vi "RCMEditor.vi"() -> ()   [LabVIEW 2020]
uses:
  <vilib>/Utility/miscctls.llb/LVSelectionTypeDef.ctl
  Type Definitions/RCMControlStatus.ctl
  Support/Tree Control/Library/TreeControl.lvclass
  Support/Refnum/Library/Refnum.lvlib
panel:
  in  "item type":string(combo)="User" caption="Item Type:"
  in  "btn1: exit":bool
  in  "btn1: save as":bool
  in  "btn1: save":bool
  in  "btn1: open":bool
  in  "btn1: new":bool
  in  "item icon path":path caption="Item ICON Path:"
  in  "item name":string caption="Item Name:"
  in  "btn2: down":bool
  in  "btn2: up":bool
  in  "btn2: indent":bool
  in  "btn2: outdent":bool
  in  "btn2: delete":bool
  in  "btn2: add":bool
  in  "tree":string(tree)
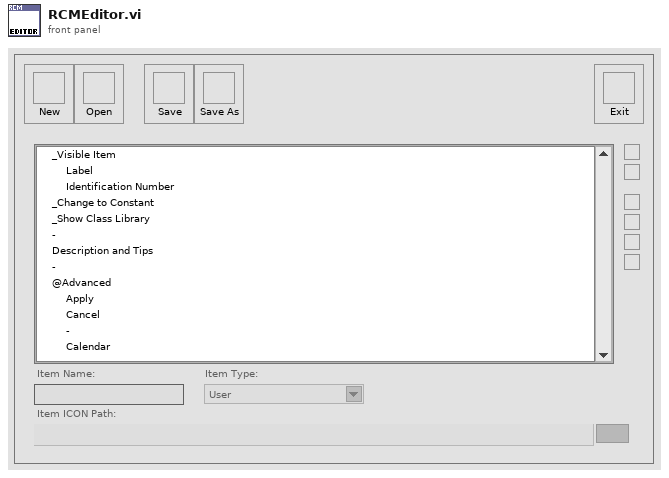
[diagram p1: front panel]
types:
  T1 = typedef "LVSelectionTypeDef.ctl" = cluster{"Selection Start":u32, "Selection End":u32}
  T2 = typedef "RCMControlStatus.ctl" = enum16{"disable all", "initialize", "enable save", "disable save", "enable tree edit", "disable tree edit", "enable item edit", "disable item edit", "user", "seperator"}
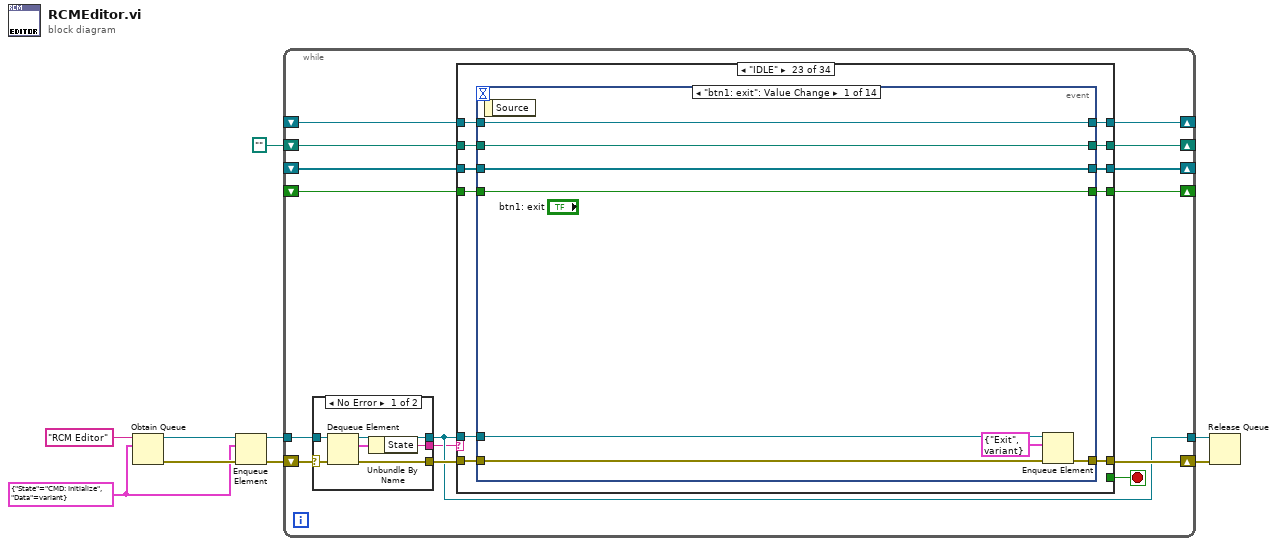
[diagram p0: block diagram]
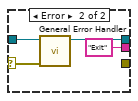
[diagram p2: hidden frame]
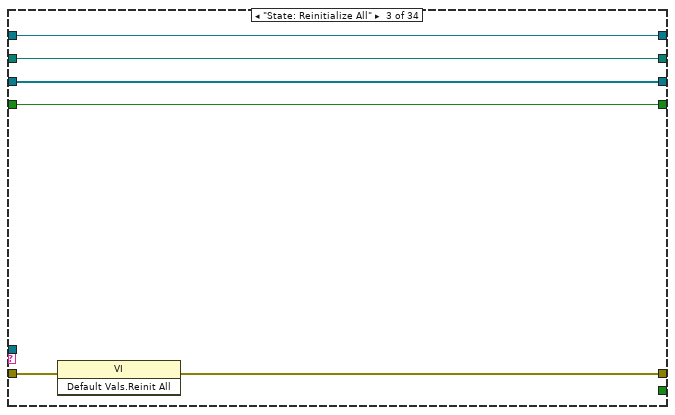
[diagram p5: hidden frame]
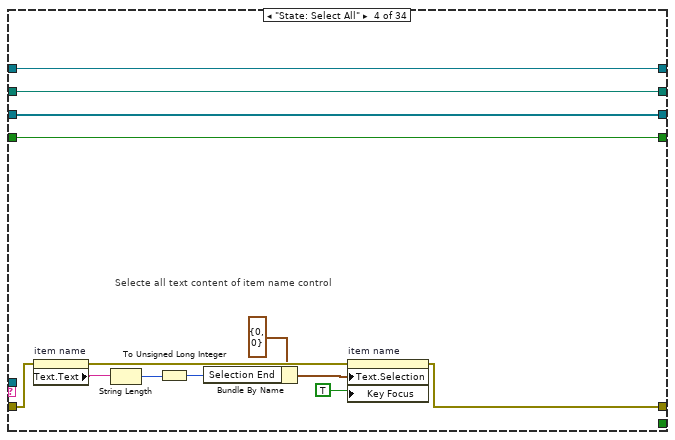
[diagram p6: hidden frame]
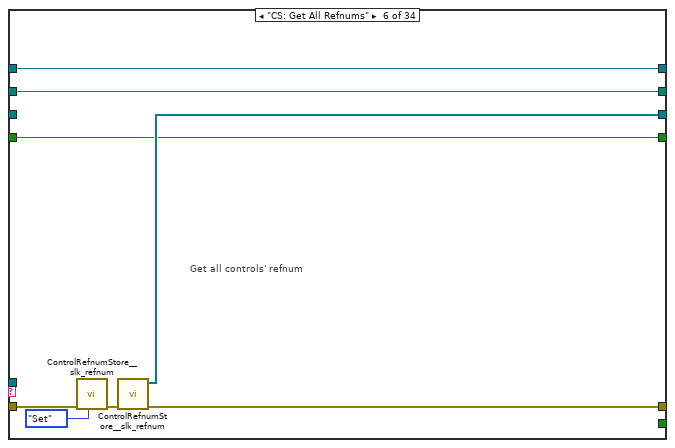
[diagram p8: hidden frame]
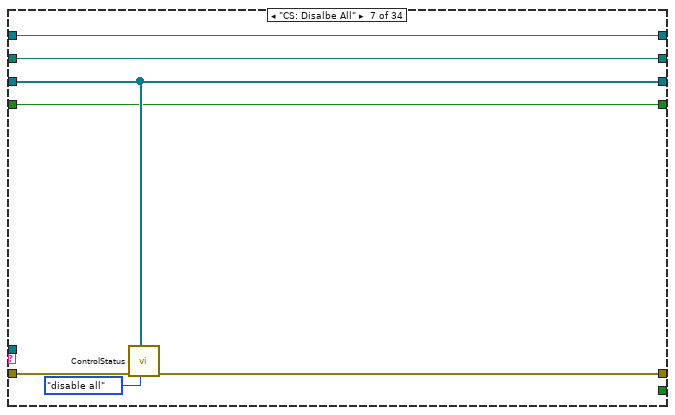
[diagram p9: hidden frame]
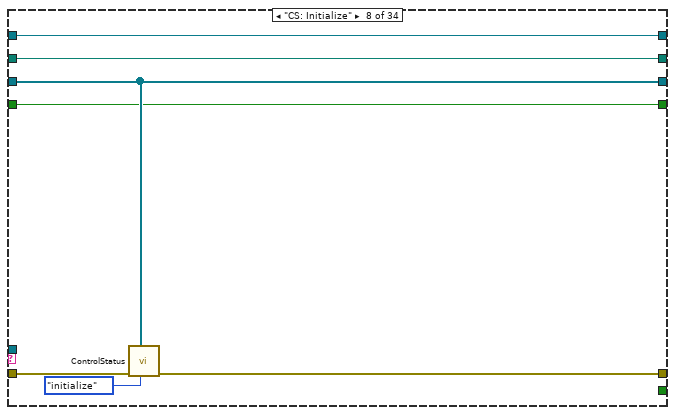
[diagram p10: hidden frame]
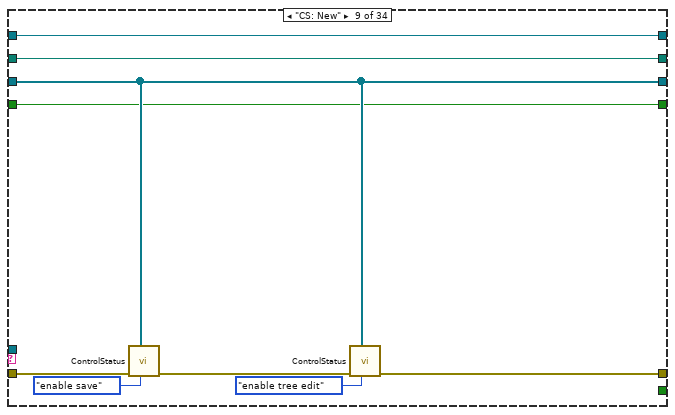
[diagram p11: hidden frame]
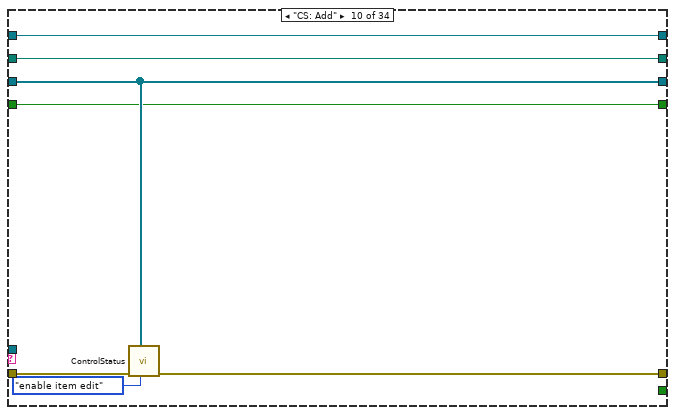
[diagram p12: hidden frame]
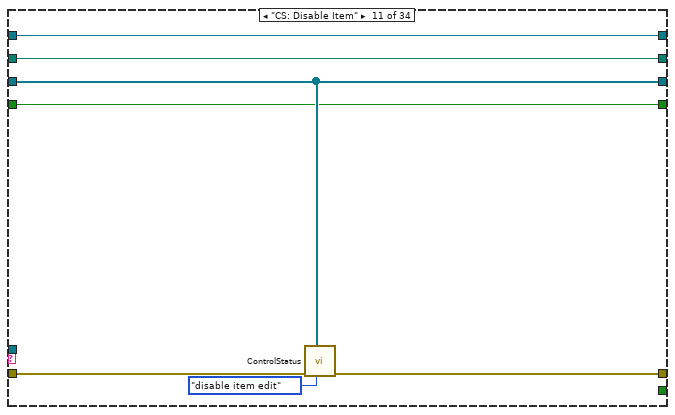
[diagram p13: hidden frame]
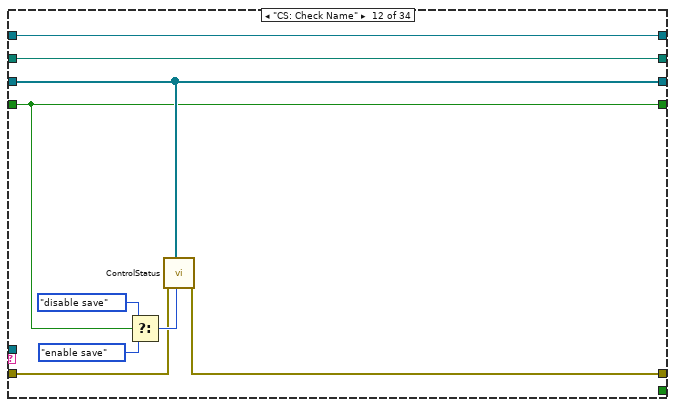
[diagram p14: hidden frame]
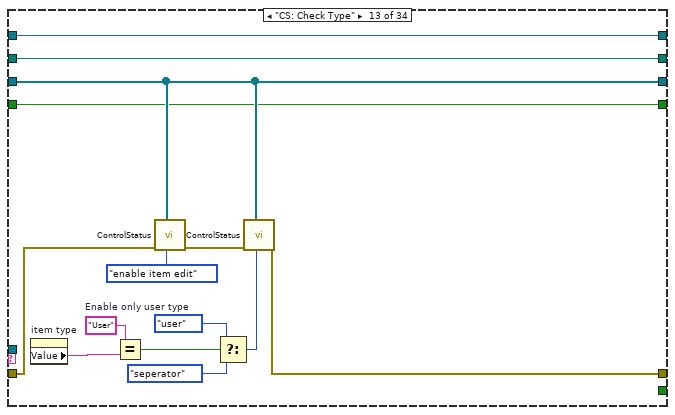
[diagram p15: hidden frame]
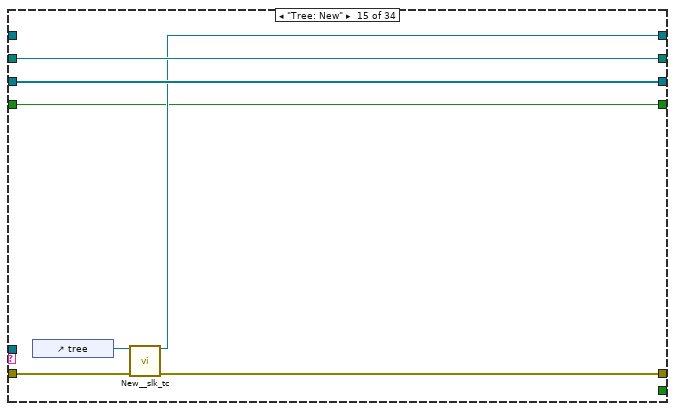
[diagram p17: hidden frame]
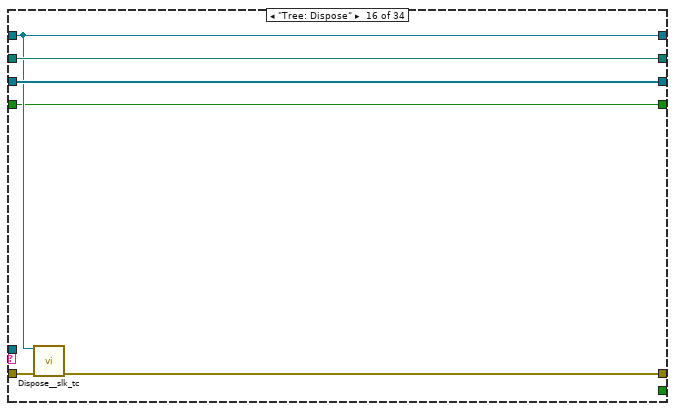
[diagram p18: hidden frame]
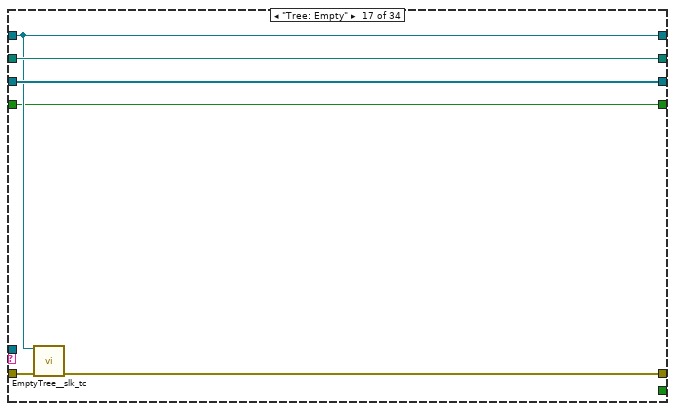
[diagram p19: hidden frame]
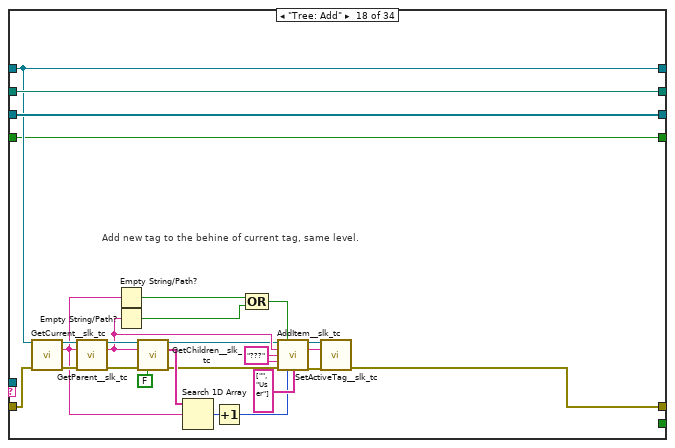
[diagram p20: hidden frame]
diagram:
  w2 = cluster{"State":string, "Data":variant} {"State"="CMD: Initialize", "Data"=variant}
  n1 = Obtain Queue(name (unnamed)="RCM Editor", element data type=w2) -> (queue out=w8:refnum<queue>, error out=w7:errorcluster)  [unwired: 3 in, 1 out]
  n2 = Enqueue Element(queue=w8, element=w2, error in (no error)=w7) -> (queue out=w4:refnum<queue>, error out=w3:errorcluster)  [unwired: 2 out]
  n3 = while {
    tunnel: w4 -> [w23]
    shift-right: [w21] -> w5
    shift-left: w3 -> [w24]
    shift-right: [w19] -> _
    shift-left: _ -> [w20]
    shift-right: [w15] -> _
    shift-left: path "" -> [w18]
    shift-right: [w16] -> _
    shift-left: _ -> [w17]
    tunnel: [w14] -> w6
    shift-right: [w11] -> _
    shift-left: _ -> [w10]
    stop <- w13 stop-if-true
    n4 = case shown="No Error" w24 {
      selector: w24 -> [w29 w33]
      tunnel: w23 -> [w30 w32]
      tunnel: [w25 "Exit" ("State")] -> w12
      tunnel: [w27 _] -> w22
      tunnel: [w26 w32] -> w14
      frame No Error {
        n5 = Dequeue Element(queue=w30, error in (no error)=w29) -> (queue out=w26:refnum<queue>, element=w28:cluster{"State":string, "Data":variant}, error out=w27:errorcluster)  [unwired: 2 out]
        n6 = Unbundle By Name(w28) -> ("State"=w25:string)
      }
      frame Error {
        n7 = call <vilib>:"General Error Handler.vi"("error in (no error)"=w33) -> ()  [unwired: 2 in, 13 out]
      }
    }
    n8 = case shown="\"IDLE\"" w12 {
      tunnel: w22 -> [w38 w43 w49 w62 w64 w72 w80 w87 w96 w103 w110 w114 w124 w140 w145 w151 w159 w173 w202 w209 w225 w242 w252 w387 w395 w407 w419 w431 w443 w455 w467 w479 w488 w491]
      tunnel: [w38 w43 w45 w50 w64 w71 w77 w84 w94 w100 w107 w113 w127 w140 w144 w150 w156 w160 w194 w206 w224 w242 w251 w387 w391 w403 w415 w427 w439 w451 w463 w475 w488 w491] -> w21
      tunnel: w14 -> [_ _ _ _ _ _ _ _ _ _ _ _ _ _ _ _ _ _ _ _ _ _ w253 _ w390 w402 w414 w426 w438 w450 w462 w474 _ _]
      tunnel: w20 -> [w37 w42 w48 w61 w67 w75 w82 w89 w98 w105 w112 w121 w128 w139 _ w149 w155 w172 w203 w208 w227 w241 w250 w386 w394 w406 w418 w430 w442 w454 w466 w478 w487 w494]
      tunnel: [w37 w42 w48 w61 w67 w75 w82 w89 w98 w105 w112 w121 w128 w139 w142 w149 w155 w172 w203 w208 w227 w241 w249 w386 w394 w406 w418 w430 w442 w454 w466 w478 w487 w494] -> w19
      tunnel: w18 -> [w35 w40 w47 w60 w66 w74 w81 w88 w97 w104 w111 w120 w135 w137 w146 w152 w157 w185 w204 w216 w237 w239 w248 w384 w392 w404 w416 w428 w440 w452 w464 w476 w485 w492]
      tunnel: w17 -> [w36 w41 w46 w59 w65 _ w79 w86 w93 w102 w109 w116 w125 w138 w147 w153 w158 w184 w205 w210 w226 w240 w247 w385 w393 w405 w417 w429 w441 w453 w465 w477 w486 w493]
      tunnel: [w36 w41 w46 w59 w65 w70 w79 w86 w93 w102 w109 w116 w125 w138 w147 w153 w158 w184 w205 w210 w226 w240 w246 w385 w393 w405 w417 w429 w441 w453 w465 w477 w486 w493] -> w16
      tunnel: [w35 w40 w47 w60 w66 w74 w81 w88 w97 w104 w111 w120 w135 w137 w146 w152 w157 w185 w204 w216 w237 w239 w245 w384 w392 w404 w416 w428 w440 w452 w464 w476 w485 w492] -> w15
      tunnel: [_ _ _ _ _ _ _ _ _ _ _ _ _ _ _ _ _ _ _ _ _ _ _ _ _ _ _ _ _ _ _ _ _ TRUE] -> w13
      tunnel: [w34 w39 w44 w58 w63 w68 w76 w83 w90 w99 w106 w115 w122 w136 w141 w148 w154 w161 w191 w207 w223 w238 w243 w383 w388 w400 w412 w424 w436 w448 w460 w472 w484 w489] -> w11
      tunnel: w10 -> [w34 w39 w44 w58 w63 w68 w76 w83 w90 w99 w106 w115 w122 w136 w141 w148 w154 w161 w191 _ w223 w238 w244 w383 w388 w400 w412 w424 w436 w448 w460 w472 w484 w489]
      frame Default {
      }
      frame "----State----" {
      }
      frame "State: Reinitialize All" {
        n9 = invoke class="VI" method="Default Vals.Reinit All"(error in=w49) -> (error out=w45:errorcluster)  [unwired: 2 in, 2 out]
      }
      frame "State: Select All" {
        # "Selecte all text content of item name control"
        n10 = property on="item name" class="Str"(error in=w62) -> (error out=w57:errorcluster, "Text.Text"=w53:string)  [unwired: 1 in, 1 out]
        n11 = String Length(string=w53) -> (length=w52:i32)
        n12 = To Unsigned Long Integer(number=w52) -> (unsigned 32bit integer=w51:u32)
        n13 = Bundle By Name(cluster=T1 {"Selection Start"=0, "Selection End"=0} ("Text.Selection"), "Selection End"=w51) -> (w54:T1)
        n14 = property on="item name" class="Str"(error in=w57, "Text.Selection"=w54, "Key Focus"=TRUE) -> (error out=w50:errorcluster)  [unwired: 1 in, 1 out]
      }
      frame "----Control Status----" {
      }
      frame "CS: Get All Refnums" {
        # "Get all controls' refnum"
        n15 = call "ControlRefnumStore__slk_refnum.vi"("cmd (Get)"=enum16{"Set", "Get"}."Set", "error in (no error)"=w72) -> ("error out"=w73:errorcluster)  [unwired: 8 in, 1 out]
        n16 = call "ControlRefnumStore__slk_refnum.vi"("error in (no error)"=w73) -> ("error out"=w71:errorcluster, "control refnum array out"=w70:refnum<vi>[])  [unwired: 9 in]
      }
      frame "CS: Disalbe All" {
        n17 = call "ControlStatus.vi"("state"=RCMControlStatus."disable all", "control refnum array in"=w79, "error in (no error)"=w80) -> ("error out"=w77:errorcluster)  [unwired: 8 in]
      }
      frame "CS: Initialize" {
        n18 = call "ControlStatus.vi"("state"=RCMControlStatus."initialize", "control refnum array in"=w86, "error in (no error)"=w87) -> ("error out"=w84:errorcluster)  [unwired: 8 in]
      }
      frame "CS: New" {
        n19 = call "ControlStatus.vi"("state"=RCMControlStatus."enable save", "control refnum array in"=w93, "error in (no error)"=w96) -> ("error out"=w95:errorcluster)  [unwired: 8 in]
        n20 = call "ControlStatus.vi"("state"=RCMControlStatus."enable tree edit", "control refnum array in"=w93, "error in (no error)"=w95) -> ("error out"=w94:errorcluster)  [unwired: 8 in]
      }
      frame "CS: Add" {
        n21 = call "ControlStatus.vi"("state"=RCMControlStatus."enable item edit", "control refnum array in"=w102, "error in (no error)"=w103) -> ("error out"=w100:errorcluster)  [unwired: 8 in]
      }
      frame "CS: Disable Item" {
        n22 = call "ControlStatus.vi"("state"=RCMControlStatus."disable item edit", "control refnum array in"=w109, "error in (no error)"=w110) -> ("error out"=w107:errorcluster)  [unwired: 8 in]
      }
      frame "CS: Check Name" {
        n23 = Select(t=RCMControlStatus."disable save" ("state"), s=w115, f=RCMControlStatus."enable save" ("state")) -> (s? t:f=w117:T2)
        n24 = call "ControlStatus.vi"("state"=w117, "control refnum array in"=w116, "error in (no error)"=w114) -> ("error out"=w113:errorcluster)  [unwired: 8 in]
      }
      frame "CS: Check Type" {
        w133 = "User"  # Enable only user type
        n25 = property on="item type" class="CmbBox"() -> ("Value"=w134:string)  [unwired: 2 in, 2 out]
        n26 = Equal?(x=w133, y=w134) -> (x = y?=w129:bool)
        n27 = call "ControlStatus.vi"("state"=RCMControlStatus."enable item edit", "control refnum array in"=w125, "error in (no error)"=w124) -> ("error out"=w123:errorcluster)  [unwired: 8 in]
        n28 = Select(t=RCMControlStatus."user" ("state"), s=w129, f=RCMControlStatus."seperator" ("state")) -> (s? t:f=w130:T2)
        n29 = call "ControlStatus.vi"("state"=w130, "control refnum array in"=w125, "error in (no error)"=w123) -> ("error out"=w127:errorcluster)  [unwired: 8 in]
      }
      frame "----Tree----" {
      }
      frame "Tree: New" {
        n30 = control-ref of="tree"() -> (w143:refnum<vi>)
        n31 = call "New__slk_tc.vi"("tree refnum"=w143, "error in (no error)"=w145) -> ("tree control out"=w142:refnum<class "TreeControl.lvclass">, "error out"=w144:errorcluster)  [unwired: 12 in]
      }
      frame "Tree: Dispose" {
        n32 = call "Dispose__slk_tc.vi"("tree control in"=w149, "error in (no error)"=w151) -> ("error out"=w150:errorcluster)  [unwired: 13 in]
      }
      frame "Tree: Empty" {
        n33 = call "EmptyTree__slk_tc.vi"("tree control in"=w155, "error in (no error)"=w159) -> ("error out"=w156:errorcluster)  [unwired: 11 in, 2 out]
      }
      frame "Tree: Add" {
        w178 = "???" ("new tag (same as text)")
        # "Add new tag to the behine of current tag, same level."
        n34 = call "GetCurrent__slk_tc.vi"("tree control in"=w172, "error in (no error)"=w173) -> ("tree control out"=w183:refnum<class "TreeControl.lvclass">, "current tag"=w168:string, "error out"=w181:errorcluster)  [unwired: 10 in, 1 out]
        n35 = call "GetParent__slk_tc.vi"("tree control in"=w183, "child tag (\"\")"=w168, "error in (no error)"=w181) -> ("tree control out"=w171:refnum<class "TreeControl.lvclass">, "parent tag"=w170:string, "error out"=w163:errorcluster)  [unwired: 9 in, 1 out]
        n36 = Empty String/Path?(string/path=w168) -> (empty?=w182:bool)
        n37 = Empty String/Path?(string/path=w170) -> (empty?=w179:bool)
        n38 = call "GetChildren__slk_tc.vi"("tree control in"=w171, "parent tag (\"\")"=w170, "error in (no error)"=w163, "use current (T)"=FALSE) -> ("tree control out"=w164:refnum<class "TreeControl.lvclass">, "children tags"=w169:string[], "error out"=w162:errorcluster)  [unwired: 9 in]
        n39 = Search 1D Array(1D array=w169, element=w168) -> (index of element=w167:i32)  [unwired: 1 in]
        n40 = Increment(x=w167) -> (x+1=w165:i32)
        n41 = Compound Arithmetic op=OR(w182, w179) -> (w180:bool)
        n42 = call "AddItem__slk_tc.vi"("tree control in"=w164, "make top level? (F)"=w180, "parent tag (current tag)"=w170, "new tag (same as text)"=w178, "new text"=w178, "error in (no error)"=w162, "child position (end=-1)"=w165, "column text {#1 and greater} (empty)"=string[] ["", "User"]) -> ("tree control out"=w177:refnum<class "TreeControl.lvclass">, "created tag"=w176:string, "error out"=w175:errorcluster)  [unwired: 5 in]
        n43 = call "SetActiveTag__slk_tc.vi"("tree control in"=w177, "active tag"=w176, "error in (no error)"=w175) -> ("error out"=w160:errorcluster)  [unwired: 11 in, 1 out]
      }
      frame "Tree: Get Value" {
        # "Ignore default value \"???\""
        n44 = call "GetCurrent__slk_tc.vi"("tree control in"=w203, "error in (no error)"=w202) -> ("tree control out"=w201:refnum<class "TreeControl.lvclass">, "current text"=w188:string, "error out"=w198:errorcluster)  [unwired: 10 in, 1 out]
        n45 = Not Equal?(x=w188, y="???" ("x")) -> (x != y?=w190:bool)
        n46 = call "GetCurrent__slk_tc.vi"("tree control in"=w201, "error in (no error)"=w198, "column # (0)"=1) -> ("tree control out"=w200:refnum<class "TreeControl.lvclass">, "current text"=w196:string, "error out"=w197:errorcluster)  [unwired: 9 in, 1 out]
        n47 = Select(t=w188, s=w190, f="") -> (s? t:f=w186:string)
        n48 = String To Path(string=w196) -> (path=w195:path)
        n49 = property on="item name" class="Str"("Value"=w186) -> ()  [unwired: 2 in, 2 out]
        n50 = property on="item icon path" class="Path"("Value"=w195) -> ()  [unwired: 2 in, 2 out]
        n51 = call "GetCurrent__slk_tc.vi"("tree control in"=w200, "error in (no error)"=w197, "column # (0)"=2) -> ("current text"=w193:string, "error out"=w194:errorcluster)  [unwired: 9 in, 2 out]
        n52 = property on="item type" class="CmbBox"("Value"=w193) -> ()  [unwired: 2 in, 2 out]
      }
      frame "Tree: Check Name" {
        # "Check if there are duplicated item name."
        n53 = call "GetAll__slk_tc.vi"("tree control in"=w208, "error in (no error)"=w209) -> ("tree control out"=w215:refnum<class "TreeControl.lvclass">, "output tree items"=w213:string[], "error out"=w214:errorcluster)  [unwired: 10 in, 1 out]
        n54 = for {
          shift-right: [w221] -> _
          shift-left: w215 -> [w222]
          tunnel: [w220] -> w212 mode=indexing
          tunnel: w213 -> [w218] mode=indexing
          shift-right: [w217] -> w211
          shift-left: w214 -> [w219]
          n55 = call "ConvertTag__slk_tc.vi"("tree control in"=w222, "input tag (current tag)"=w218, "error in (no error)"=w219) -> ("tree control out"=w221:refnum<class "TreeControl.lvclass">, "text"=w220:string, "error out"=w217:errorcluster)  [unwired: 9 in, 1 out]
        }
        n56 = call "CheckName.vi"("error in (no error)"=w211, "input array"=w212) -> ("error out"=w206:errorcluster, "duplicated?"=w207:bool)  [unwired: 8 in]
      }
      frame "Tree: Type Change" {
        n57 = call "EditItem__slk_tc.vi"("tree control in"=w227, "new text"="-", "error in (no error)"=w225) -> ("tree control out"=w235:refnum<class "TreeControl.lvclass">, "error out"=w234:errorcluster)  [unwired: 11 in]
        n58 = call "EditItem__slk_tc.vi"("tree control in"=w235, "new text"="", "error in (no error)"=w234, "column # (0)"=1) -> ("tree control out"=w231:refnum<class "TreeControl.lvclass">, "error out"=w230:errorcluster)  [unwired: 10 in]
        n59 = property on="item type" class="CmbBox"() -> ("Value"=w228:string)  [unwired: 2 in, 2 out]
        n60 = call "EditItem__slk_tc.vi"("tree control in"=w231, "new text"=w228, "error in (no error)"=w230, "column # (0)"=2) -> ("error out"=w224:errorcluster)  [unwired: 10 in, 1 out]
      }
      frame "----Event----" {
      }
      frame "IDLE" {
        n61 = event shown="[0] \"btn1: exit\": Value Change" {
          selector: _ -> [_ _ _ _ _ _ _ _ _ _ _ _ _ _]
          dyn-events: _ -> [_ _ _ _ _ _ _ _ _ _ _ _ _ _]
          timeout: _ -> [_ _ _ _ _ _ _ _ _ _ _ _ _ _]
          tunnel: w253 -> [w256 w264 w271 w283 w292 w301 w310 w319 w327 w342 w351 w362 w372 w381]
          tunnel: w252 -> [w257 w265 w272 w280 w289 w298 w307 w316 w324 w333 w347 w358 w368 w375]
          tunnel: [w261 w269 w277 w286 w295 w304 w313 w322 w330 w345 w353 w363 w373 w382] -> w251
          tunnel: w250 -> [w260 w268 w273 w281 w290 w299 w308 w317 w325 w335 w349 w359 w369 w378]
          tunnel: [w260 w268 w273 w281 w290 w299 w308 w317 w325 w335 w349 w359 w369 w378] -> w249
          tunnel: w248 -> [w259 w267 w276 w285 w294 w303 w312 w321 w329 w344 w352 w356 _ _]
          tunnel: w247 -> [w258 w266 w275 w284 w293 w302 w311 w320 w328 w343 w348 w360 w370 w379]
          tunnel: [w258 w266 w275 w284 w293 w302 w311 w320 w328 w343 w348 w360 w370 w379] -> w246
          tunnel: [w259 w267 w276 w285 w294 w303 w312 w321 w329 w344 w352 w355 w366 w377] -> w245
          tunnel: w244 -> [w254 w262 w270 w278 w287 w296 w305 w314 w323 w331 w346 w354 w364 w376]
          tunnel: [w254 w262 w270 w278 w287 w296 w305 w314 w323 w331 w346 w354 w364 w376] -> w243
          event "btn1: exit": Value Change {
            n62 = event-data() -> ()  [unwired: 2 out]
            n63 = Enqueue Element(queue=w256, element=cluster{"State":string, "Data":variant} {"State"="Exit", "Data"=variant}, error in (no error)=w257) -> (error out=w261:errorcluster)  [unwired: 3 out]
          }
          event "btn1: new": Value Change {
            n64 = event-data() -> ()  [unwired: 2 out]
            n65 = Enqueue Element(queue=w264, element=cluster{"State":string, "Data":variant} {"State"="CMD: New", "Data"=variant}, error in (no error)=w265) -> (error out=w269:errorcluster)  [unwired: 3 out]
          }
          event "btn2: add": Value Change {
            n66 = event-data() -> ()  [unwired: 2 out]
            n67 = Enqueue Element(queue=w271, element=cluster{"State":string, "Data":variant} {"State"="CMD: Add", "Data"=variant}, error in (no error)=w272) -> (error out=w277:errorcluster)  [unwired: 3 out]
          }
          event "btn2: delete": Value Change {
            n68 = event-data() -> ()  [unwired: 2 out]
            n69 = call "RemoveItem__slk_tc.vi"("tree control in"=w281, "error in (no error)"=w280) -> ("error out"=w279:errorcluster)  [unwired: 12 in, 1 out]
            n70 = Enqueue Element(queue=w283, element=cluster{"State":string, "Data":variant} {"State"="CMD: Delete", "Data"=variant}, error in (no error)=w279) -> (error out=w286:errorcluster)  [unwired: 3 out]
          }
          event "btn2: outdent": Value Change {
            n71 = event-data() -> ()  [unwired: 2 out]
            n72 = call "OutdentItem__slk_tc.vi"("tree control in"=w290, "error in (no error)"=w289) -> ("error out"=w288:errorcluster)  [unwired: 12 in, 1 out]
            n73 = Enqueue Element(queue=w292, element=cluster{"State":string, "Data":variant} {"State"="IDLE", "Data"=variant}, error in (no error)=w288) -> (error out=w295:errorcluster)  [unwired: 3 out]
          }
          event "btn2: indent": Value Change {
            n74 = event-data() -> ()  [unwired: 2 out]
            n75 = call "IndentItem__slk_tc.vi"("tree control in"=w299, "error in (no error)"=w298) -> ("error out"=w297:errorcluster)  [unwired: 12 in, 1 out]
            n76 = Enqueue Element(queue=w301, element=cluster{"State":string, "Data":variant} {"State"="IDLE", "Data"=variant}, error in (no error)=w297) -> (error out=w304:errorcluster)  [unwired: 3 out]
          }
          event "btn2: up": Value Change {
            n77 = event-data() -> ()  [unwired: 2 out]
            n78 = call "UpItem__slk_tc.vi"("tree control in"=w308, "error in (no error)"=w307) -> ("error out"=w306:errorcluster)  [unwired: 12 in, 1 out]
            n79 = Enqueue Element(queue=w310, element=cluster{"State":string, "Data":variant} {"State"="IDLE", "Data"=variant}, error in (no error)=w306) -> (error out=w313:errorcluster)  [unwired: 3 out]
          }
          event "btn2: down": Value Change {
            n80 = event-data() -> ()  [unwired: 2 out]
            n81 = call "DownItem__slk_tc.vi"("tree control in"=w317, "error in (no error)"=w316) -> ("error out"=w315:errorcluster)  [unwired: 12 in, 1 out]
            n82 = Enqueue Element(queue=w319, element=cluster{"State":string, "Data":variant} {"State"="IDLE", "Data"=variant}, error in (no error)=w315) -> (error out=w322:errorcluster)  [unwired: 3 out]
          }
          event "tree": Value Change {
            n83 = event-data() -> ()  [unwired: 2 out]
            n84 = Enqueue Element(queue=w327, element=cluster{"State":string, "Data":variant} {"State"="CMD: Tree Value Change", "Data"=variant}, error in (no error)=w324) -> (error out=w330:errorcluster)  [unwired: 3 out]
          }
          event "item name", "item icon path": Value Change {
            n85 = event-data() -> ()  [unwired: 2 out]
            n86 = property on="item name" class="Str"() -> ("Value"=w337:string)  [unwired: 2 in, 2 out]
            n87 = call "EditItem__slk_tc.vi"("tree control in"=w335, "new text"=w337, "error in (no error)"=w333) -> ("tree control out"=w336:refnum<class "TreeControl.lvclass">, "error out"=w334:errorcluster)  [unwired: 11 in]
            n88 = property on="item icon path" class="Path"() -> ("Value"=w340:path)  [unwired: 2 in, 2 out]
            n89 = Path To String(path=w340) -> (string=w338:string)
            n90 = call "EditItem__slk_tc.vi"("tree control in"=w336, "new text"=w338, "error in (no error)"=w334, "column # (0)"=1) -> ("error out"=w332:errorcluster)  [unwired: 10 in, 1 out]
            n91 = Enqueue Element(queue=w342, element=cluster{"State":string, "Data":variant} {"State"="CMD: Value Change", "Data"=variant}, error in (no error)=w332) -> (error out=w345:errorcluster)  [unwired: 3 out]
          }
          event "item type": Value Change {
            n92 = event-data() -> ()  [unwired: 2 out]
            n93 = Enqueue Element(queue=w351, element=cluster{"State":string, "Data":variant} {"State"="CMD: Type Change", "Data"=variant}, error in (no error)=w347) -> (error out=w353:errorcluster)  [unwired: 3 out]
          }
          event "btn1: save": Value Change {
            n94 = event-data() -> ()  [unwired: 2 out]
            n95 = call "WriteTreeToRCMFile.vi"("tree control"=w359, "error in (no error)"=w358, "rcm file path in"=w356) -> ("error out"=w357:errorcluster, "rcm file path out"=w355:path)  [unwired: 7 in]
            n96 = Enqueue Element(queue=w362, element=cluster{"State":string, "Data":variant} {"State"="IDLE", "Data"=variant}, error in (no error)=w357) -> (error out=w363:errorcluster)  [unwired: 3 out]
          }
          event "btn1: save as": Value Change {
            n97 = event-data() -> ()  [unwired: 2 out]
            n98 = call "WriteTreeToRCMFile.vi"("tree control"=w369, "error in (no error)"=w368, "rcm file path in"=path "") -> ("error out"=w367:errorcluster, "rcm file path out"=w366:path)  [unwired: 7 in]
            n99 = Enqueue Element(queue=w372, element=cluster{"State":string, "Data":variant} {"State"="IDLE", "Data"=variant}, error in (no error)=w367) -> (error out=w373:errorcluster)  [unwired: 3 out]
          }
          event "btn1: open": Value Change {
            n100 = event-data() -> ()  [unwired: 2 out]
            n101 = call "ReadRCMFileToTree.vi"("tree control"=w378, "error in (no error)"=w375) -> ("error out"=w374:errorcluster, "rcm file path out"=w377:path)  [unwired: 8 in]
            n102 = Enqueue Element(queue=w381, element=cluster{"State":string, "Data":variant} {"State"="CMD: Open", "Data"=variant}, error in (no error)=w374) -> (error out=w382:errorcluster)  [unwired: 3 out]
          }
        }
      }
      frame "----Command----" {
      }
      frame "CMD: Initialize" {
        n103 = for {
          tunnel: w390 -> [w397]
          shift-right: [w398] -> w391
          shift-left: w395 -> [w399]
          tunnel: cluster{"State":string, "Data":variant}[] [{"State"="State: Reinitialize All", "Data"=variant}, {"State"="CS: Get All Refnums", "Data"=variant}, {"State"="CS: Disalbe All", "Data"=variant}, {"State"="CS: Initialize", "Data"=variant}, {"State"="Tree: New", "Data"=variant}, {"State"="Tree: Empty", "Data"=variant}, {"State"="IDLE", "Data"=variant}] -> [w396] mode=indexing
          n104 = Enqueue Element(queue=w397, element=w396, error in (no error)=w399) -> (error out=w398:errorcluster)  [unwired: 1 in, 2 out]
        }
      }
      frame "CMD: New" {
        n105 = for {
          tunnel: w402 -> [w409]
          shift-right: [w410] -> w403
          shift-left: w407 -> [w411]
          tunnel: cluster{"State":string, "Data":variant}[] [{"State"="State: Reinitialize All", "Data"=variant}, {"State"="CS: New", "Data"=variant}, {"State"="Tree: New", "Data"=variant}, {"State"="Tree: Empty", "Data"=variant}, {"State"="IDLE", "Data"=variant}] -> [w408] mode=indexing
          n106 = Enqueue Element(queue=w409, element=w408, error in (no error)=w411) -> (error out=w410:errorcluster)  [unwired: 1 in, 2 out]
        }
      }
      frame "CMD: Add" {
        n107 = for {
          tunnel: w414 -> [w421]
          shift-right: [w422] -> w415
          shift-left: w419 -> [w423]
          tunnel: cluster{"State":string, "Data":variant}[] [{"State"="CS: Add", "Data"=variant}, {"State"="Tree: Add", "Data"=variant}, {"State"="State: Select All", "Data"=variant}, {"State"="Tree: Get Value", "Data"=variant}, {"State"="Tree: Check Name", "Data"=variant}, {"State"="CS: Check Name", "Data"=variant}, {"State"="IDLE", "Data"=variant}] -> [w420] mode=indexing
          n108 = Enqueue Element(queue=w421, element=w420, error in (no error)=w423) -> (error out=w422:errorcluster)  [unwired: 1 in, 2 out]
        }
      }
      frame "CMD: Open" {
        n109 = for {
          tunnel: w426 -> [w433]
          shift-right: [w434] -> w427
          shift-left: w431 -> [w435]
          tunnel: cluster{"State":string, "Data":variant}[] [{"State"="CS: New", "Data"=variant}, {"State"="CS: Disable Item", "Data"=variant}, {"State"="IDLE", "Data"=variant}] -> [w432] mode=indexing
          n110 = Enqueue Element(queue=w433, element=w432, error in (no error)=w435) -> (error out=w434:errorcluster)  [unwired: 1 in, 2 out]
        }
      }
      frame "CMD: Value Change" {
        n111 = for {
          tunnel: w438 -> [w445]
          shift-right: [w446] -> w439
          shift-left: w443 -> [w447]
          tunnel: cluster{"State":string, "Data":variant}[] [{"State"="Tree: Get Value", "Data"=variant}, {"State"="Tree: Check Name", "Data"=variant}, {"State"="CS: Check Name", "Data"=variant}, {"State"="CS: Check Type", "Data"=variant}, {"State"="IDLE", "Data"=variant}] -> [w444] mode=indexing
          n112 = Enqueue Element(queue=w445, element=w444, error in (no error)=w447) -> (error out=w446:errorcluster)  [unwired: 1 in, 2 out]
        }
      }
      frame "CMD: Tree Value Change" {
        n113 = for {
          tunnel: w450 -> [w457]
          shift-right: [w458] -> w451
          shift-left: w455 -> [w459]
          tunnel: cluster{"State":string, "Data":variant}[] [{"State"="Tree: Get Value", "Data"=variant}, {"State"="State: Select All", "Data"=variant}, {"State"="Tree: Check Name", "Data"=variant}, {"State"="CS: Check Name", "Data"=variant}, {"State"="CS: Check Type", "Data"=variant}, {"State"="IDLE", "Data"=variant}] -> [w456] mode=indexing
          n114 = Enqueue Element(queue=w457, element=w456, error in (no error)=w459) -> (error out=w458:errorcluster)  [unwired: 1 in, 2 out]
        }
      }
      frame "CMD: Delete" {
        n115 = for {
          tunnel: w462 -> [w469]
          shift-right: [w470] -> w463
          shift-left: w467 -> [w471]
          tunnel: cluster{"State":string, "Data":variant}[] [{"State"="Tree: Check Name", "Data"=variant}, {"State"="CS: Check Name", "Data"=variant}, {"State"="CS: Disable Item", "Data"=variant}, {"State"="IDLE", "Data"=variant}] -> [w468] mode=indexing
          n116 = Enqueue Element(queue=w469, element=w468, error in (no error)=w471) -> (error out=w470:errorcluster)  [unwired: 1 in, 2 out]
        }
      }
      frame "CMD: Type Change" {
        n117 = for {
          tunnel: w474 -> [w481]
          shift-right: [w482] -> w475
          shift-left: w479 -> [w483]
          tunnel: cluster{"State":string, "Data":variant}[] [{"State"="Tree: Type Change", "Data"=variant}, {"State"="CS: Check Type", "Data"=variant}, {"State"="Tree: Get Value", "Data"=variant}, {"State"="Tree: Check Name", "Data"=variant}, {"State"="CS: Check Name", "Data"=variant}, {"State"="IDLE", "Data"=variant}] -> [w480] mode=indexing
          n118 = Enqueue Element(queue=w481, element=w480, error in (no error)=w483) -> (error out=w482:errorcluster)  [unwired: 1 in, 2 out]
        }
      }
      frame "----Exit----" {
      }
      frame "Exit" {
      }
    }
  }
  n119 = Release Queue(queue=w6, error in (no error)=w5) -> ()  [unwired: 4 out]
